vi "HW_Init.vi"(8 "error in":errorcluster, 9 "Traget FPS":i32=80, 10 "Close port? (T)":bool=TRUE, 11 "VISA resource name":refnum<visa-resource-name>="ASRL3::INSTR") -> (0 "error out":errorcluster, 1 "Sensors response":string="A1454", 2 "Instrument OK?":bool=TRUE, 3 "VISA resource name out":refnum<visa-resource-name>="ASRL3::INSTR", 4 "Sync mode status":string, 5 "Sensor board size":string, 6 "FPS status":i32=80, 7 "Version information":string)   [LabVIEW 2016]
uses:
  <vilib>/Utility/error.llb/DialogType.ctl
  <vilib>/Instr/_visa.llb/VISA Set IO Buffer Mask.ctl
  <vilib>/Instr/_visa.llb/VISA Flush IO Buffer Mask.ctl
  <vilib>/Instr/_visa.llb/VISA Configure Serial Port (Instr).vi
panel:
  out "Poll Sync mode status":u32
  out "Poll Port data status":u32
  out "Port data status":i32=1
  out "Latest Poll results (before implemented adjustments)":string="P\r\nI am alive!\r\nA1454 OK!\r\nBinary mode ON\r\nCoordinate mode ON\r\nMatrix mode OFF\r\nFPS target=80\r\nExternal USART status: 0\r\nLed status: 1\r\nPort data status: 1\r\nIOS: 1 = 0, 2 = 0 3 = 0, 4 = 0\r\nOK\r\n"
  out "Poll Binary":u32
  out "Poll Matrix":u32
  out "Poll Coord":u32
  out "Poll FPS":u32
  out "Matrix mode status":string="OFF"
  out "Coordinate mode status":string="ON"
  out "Binary mode status":string="ON"
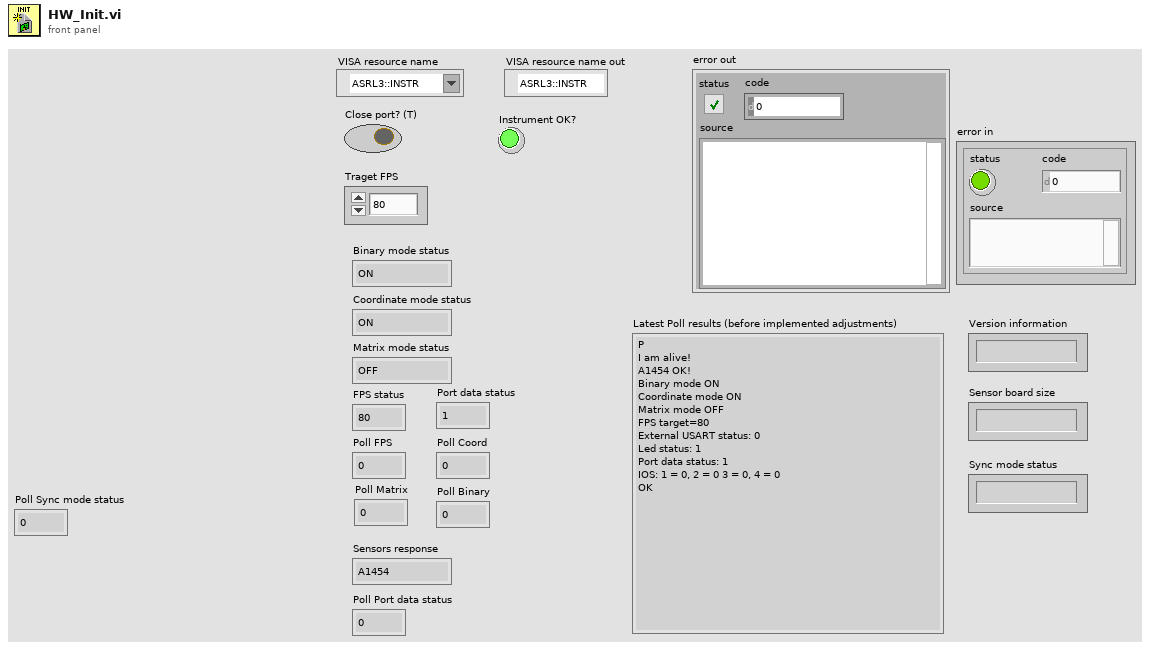
[diagram p1: front panel]
types:
  T1 = typedef "DialogType.ctl" = u16
  T2 = typedef "VISA Set IO Buffer Mask.ctl" = u16
  T3 = typedef "VISA Flush IO Buffer Mask.ctl" = u16
  T4 = cluster{"Matrix mode status":string, "Coordinate mode status":string, "Binary mode status":string, "Sensors response":string, "FPS status":i32, "Port data status":i32}
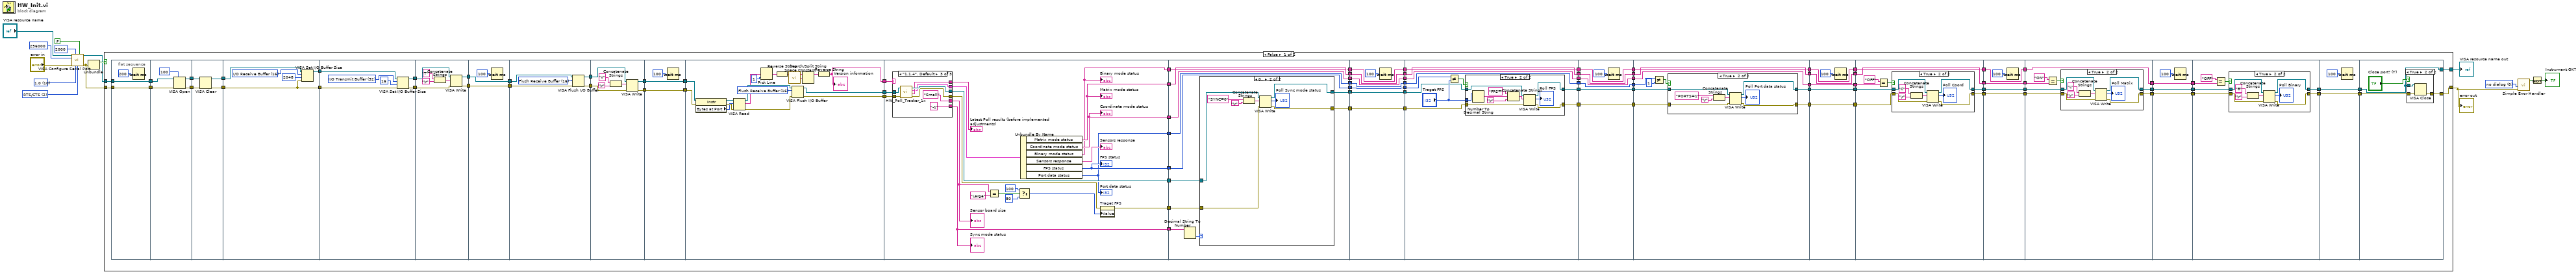
[diagram p0: block diagram]
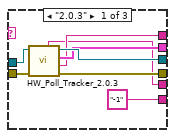
[diagram p2: hidden frame]
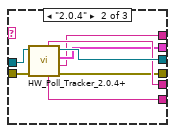
[diagram p3: hidden frame]
diagram:
  w1 = u16 10 items=["1.0"=10, "1.5"=15, "2.0"=20] ("stop bits (10: 1 bit)")
  w3 = T1 0 items=["no dialog", "OK message", "continue or stop message", "OK message + warnings", "continue/stop + warnings"] ("type of dialog (OK msg:1)")
  w9 = u16 2 items=["None", "XON/XOFF", "RTS/CTS", "XON/XOFF & RTS/CTS", "DTR/DSR", "XON/XOFF & DTR/DSR"] ("flow control (0:none)")
  n1 = call-poly "VISA Configure Serial Port"("VISA resource name"="VISA resource name", "timeout (10sec)"=u32 2000, "Enable Termination\nChar (T)"=FALSE ("Enable Termination\nChar (T)"), "baud rate (9600)"=u32 256000, "error in (no error)"="error in", "stop bits (10: 1 bit)"=w1, "flow control (0:none)"=w9) -> ("VISA resource name out"=w7:refnum<visa-resource-name>, "error out"=w11:errorcluster)  [unwired: 7 in]
  n2 = Unbundle(w11) -> ("status"=w10:bool)  [unwired: 2 out]
  n3 = case shown="False" w10 {
    tunnel: w7 -> [w73 w374]
    tunnel: w11 -> [w72 w375]
    tunnel: [w54 w375] -> w6
    tunnel: [w53 w374] -> w8
    frame False {
      n4 = flat-sequence {
        tunnel: [w106] -> w104
        tunnel: [w105] -> w103
        tunnel: w73 -> [w106]
        tunnel: w72 -> [w105]
        tunnel: w104 -> [w110]
        tunnel: [w109] -> w101
        tunnel: w103 -> [w112]
        tunnel: [w111] -> w102
        tunnel: w102 -> [w115]
        tunnel: w101 -> [w116]
        tunnel: [w114] -> w100
        tunnel: [w113] -> w99
        tunnel: [w117] -> w97
        tunnel: [w121] -> w98
        tunnel: w100 -> [w117]
        tunnel: w99 -> [w119]
        tunnel: w98 -> [w125]
        tunnel: [w124] -> w46
        tunnel: w97 -> [w123]
        tunnel: [w122] -> w45
        tunnel: w46 -> [w131]
        tunnel: [w129] -> w42
        tunnel: w45 -> [w130]
        tunnel: [w128] -> w40
        tunnel: w42 -> [w137]
        tunnel: [w137] -> w41
        tunnel: w40 -> [w136]
        tunnel: [w136] -> w39
        tunnel: w41 -> [w140]
        tunnel: [w139] -> w44
        tunnel: w39 -> [w142]
        tunnel: [w141] -> w43
        tunnel: w44 -> [w145]
        tunnel: w43 -> [w146]
        tunnel: [w144] -> w52
        tunnel: [w143] -> w51
        tunnel: w52 -> [w152]
        tunnel: [w152] -> w50
        tunnel: w51 -> [w151]
        tunnel: [w151] -> w48
        tunnel: w50 -> [w165]
        tunnel: [w163] -> w49
        tunnel: w48 -> [w166]
        tunnel: [w161] -> w47
        tunnel: [w153] -> w38
        tunnel: [w177] -> w29
        tunnel: [w190] -> w30
        tunnel: w49 -> [w188]
        tunnel: [w181] -> w27
        tunnel: [w184] -> w25
        tunnel: [w185] -> w23
        tunnel: [w183] -> w21
        tunnel: [w180] -> w19
        tunnel: w47 -> [w187]
        tunnel: w38 -> [w179]
        tunnel: [w170] -> w16
        tunnel: w30 -> [w220]
        tunnel: w29 -> [w218]
        tunnel: [w217] -> w28
        tunnel: w27 -> [w225]
        tunnel: [w225] -> w26
        tunnel: w25 -> [w224]
        tunnel: [w224] -> w24
        tunnel: w23 -> [w223]
        tunnel: [w223] -> w22
        tunnel: w21 -> [w222]
        tunnel: [w222] -> w20
        tunnel: w19 -> [w221]
        tunnel: [w221] -> w18
        tunnel: [w219] -> w17
        tunnel: w16 -> [w216]
        tunnel: [w243] -> w37
        tunnel: w28 -> [w242]
        tunnel: [w242] -> w36
        tunnel: w26 -> [w241]
        tunnel: [w241] -> w35
        tunnel: w24 -> [w240]
        tunnel: [w240] -> w34
        tunnel: w22 -> [w239]
        tunnel: [w239] -> w33
        tunnel: w20 -> [w238]
        tunnel: [w238] -> w32
        tunnel: w18 -> [w237]
        tunnel: [w237] -> w31
        tunnel: w17 -> [w243]
        tunnel: w37 -> [w252]
        tunnel: [w249] -> w96
        tunnel: w36 -> [w251]
        tunnel: [w250] -> w95
        tunnel: w35 -> [w253]
        tunnel: [w248] -> w94
        tunnel: w34 -> [w248]
        tunnel: [w247] -> w93
        tunnel: w33 -> [w247]
        tunnel: [w246] -> w92
        tunnel: w32 -> [w246]
        tunnel: w31 -> [w245]
        tunnel: [w245] -> w55
        tunnel: w96 -> [w273]
        tunnel: [w273] -> w71
        tunnel: w95 -> [w272]
        tunnel: [w272] -> w70
        tunnel: [w270] -> w69
        tunnel: w94 -> [w270]
        tunnel: [w269] -> w68
        tunnel: w93 -> [w269]
        tunnel: [w268] -> w67
        tunnel: w92 -> [w268]
        tunnel: [w267] -> w56
        tunnel: w55 -> [w267]
        tunnel: w71 -> [w278]
        tunnel: [w277] -> w66
        tunnel: w70 -> [w280]
        tunnel: [w279] -> w64
        tunnel: w69 -> [w283]
        tunnel: [w283] -> w62
        tunnel: w68 -> [w282]
        tunnel: [w282] -> w60
        tunnel: w67 -> [w281]
        tunnel: [w281] -> w58
        tunnel: w56 -> [w275]
        tunnel: w66 -> [w299]
        tunnel: [w299] -> w65
        tunnel: w64 -> [w298]
        tunnel: [w298] -> w63
        tunnel: w62 -> [w297]
        tunnel: [w297] -> w61
        tunnel: w60 -> [w296]
        tunnel: [w296] -> w59
        tunnel: w58 -> [w295]
        tunnel: [w295] -> w57
        tunnel: w65 -> [w307]
        tunnel: [w305] -> w91
        tunnel: w63 -> [w306]
        tunnel: [w302] -> w90
        tunnel: w61 -> [w304]
        tunnel: w59 -> [w301]
        tunnel: [w301] -> w89
        tunnel: w57 -> [w300]
        tunnel: [w300] -> w88
        tunnel: w91 -> [w323]
        tunnel: [w323] -> w87
        tunnel: w90 -> [w322]
        tunnel: [w322] -> w86
        tunnel: [w320] -> w85
        tunnel: w89 -> [w320]
        tunnel: [w319] -> w84
        tunnel: w88 -> [w319]
        tunnel: w87 -> [w329]
        tunnel: [w327] -> w83
        tunnel: w86 -> [w328]
        tunnel: [w326] -> w82
        tunnel: w85 -> [w325]
        tunnel: w84 -> [w324]
        tunnel: [w324] -> w81
        tunnel: w83 -> [w345]
        tunnel: [w345] -> w80
        tunnel: w82 -> [w344]
        tunnel: [w344] -> w79
        tunnel: [w342] -> w78
        tunnel: w81 -> [w342]
        tunnel: w80 -> [w350]
        tunnel: [w348] -> w77
        tunnel: w79 -> [w349]
        tunnel: [w347] -> w76
        tunnel: w78 -> [w346]
        tunnel: w77 -> [w365]
        tunnel: [w365] -> w75
        tunnel: [w364] -> w74
        tunnel: w76 -> [w364]
        tunnel: w75 -> [w366]
        tunnel: w74 -> [w369]
        tunnel: [w367] -> w54
        tunnel: [w366] -> w53
        frame #0 {
          n5 = Wait (ms)(milliseconds to wait=u32 200) -> ()  [unwired: 1 out]
        }
        frame #1 {
          n6 = VISA Open(timeout (0)=u32 100 ("VISA Open timeout (0)"), error in (no error)=w112, VISA resource name=w110) -> (VISA resource name=w109:refnum<visa-resource-name>, error out=w111:errorcluster)  [unwired: 2 in]
        }
        frame #2 {
          n7 = VISA Clear(VISA resource name=w116, error in (no error)=w115) -> (VISA resource name out=w113:refnum<visa-resource-name>, error out=w114:errorcluster)
        }
        frame #3 {
          w118 = T2 16 items=["I/O Receive Buffer"=16, "I/O Transmit Buffer"=32, "I/O Receive and Transmit Buffer"=48] ("Mask")
          n8 = VISA Set I/O Buffer Size(VISA resource name=w119, mask (16)=w118, size (4096)=u32 2048, error in (no error)=w117) -> (VISA resource name out=w121:refnum<visa-resource-name>)  [unwired: 1 out]
        }
        frame #4 {
          w126 = T2 32 items=["I/O Receive Buffer"=16, "I/O Transmit Buffer"=32, "I/O Receive and Transmit Buffer"=48] ("Mask")
          n9 = VISA Set I/O Buffer Size(VISA resource name=w125, mask (16)=w126, size (4096)=u32 16, error in (no error)=w123) -> (VISA resource name out=w124:refnum<visa-resource-name>, error out=w122:errorcluster)
        }
        frame #5 {
          n10 = Concatenate Strings("T" ("write buffer"), "\r") -> (w132:string)
          n11 = VISA Write(VISA resource name=w131, write buffer=w132, error in (no error)=w130) -> (VISA resource name out=w129:refnum<visa-resource-name>, error out=w128:errorcluster)  [unwired: 1 out]
        }
        frame #6 {
          n12 = Wait (ms)(milliseconds to wait=u32 100) -> ()  [unwired: 1 out]
        }
        frame #7 {
          w138 = T3 16 items=["Flush Receive Buffer"=16, "Write Transmit Buffer to Device"=32, "Flush Receive Buffer (No I/O)"=64, "Flush Transmit Buffer"=128] ("Mask")
          n13 = VISA Flush I/O Buffer(VISA resource name=w140, mask (16)=w138, error in (no error)=w142) -> (VISA resource name out=w139:refnum<visa-resource-name>, error out=w141:errorcluster)
        }
        frame #8 {
          n14 = Concatenate Strings("V" ("write buffer"), "\r") -> (w147:string)
          n15 = VISA Write(VISA resource name=w145, write buffer=w147, error in (no error)=w146) -> (VISA resource name out=w143:refnum<visa-resource-name>, error out=w144:errorcluster)  [unwired: 1 out]
        }
        frame #9 {
          n16 = Wait (ms)(milliseconds to wait=u32 100) -> ()  [unwired: 1 out]
        }
        frame #10 {
          w160 = T3 16 items=["Flush Receive Buffer"=16, "Write Transmit Buffer to Device"=32, "Flush Receive Buffer (No I/O)"=64, "Flush Transmit Buffer"=128] ("Mask")
          n17 = property class="Instr"(reference=w166, error in=w165) -> (reference out=w169:refnum<visa-resource-name>, error out=w168:errorcluster, "Bytes at Port"=w167:u32)
          n18 = VISA Read(VISA resource name=w169, byte count=w167, error in (no error)=w168) -> (VISA resource name out=w162:refnum<visa-resource-name>, read buffer=w159:string, error out=w164:errorcluster)  [unwired: 1 out]
          n19 = Pick Line(multi-line string=w159, line index=1) -> (output string=w157:string)  [unwired: 1 in]
          n20 = Reverse String(1:w157) -> (0:w156:string)
          n21 = call <vilib>:"Space Constant.vi"() -> ("String"=w155:string)
          n22 = VISA Flush I/O Buffer(VISA resource name=w162, mask (16)=w160, error in (no error)=w164) -> (VISA resource name out=w161:refnum<visa-resource-name>, error out=w163:errorcluster)
          n23 = Search/Split String(string=w156, search string/char (-)=w155) -> (substring before match=w154:string)  [unwired: 1 in, 2 out]
          n24 = Reverse String(1:w154) -> (0:w153:string)
          "Version information" <- w153
        }
        frame #11 {
          n25 = case shown="\"1.1.4\", Default" w179 {
            tunnel: [w195 w204 w214] -> w190
            tunnel: [w193 w201 w213] -> w189
            tunnel: w188 -> [w198 w205 w212]
            tunnel: w187 -> [w196 w206 w211]
            tunnel: [w197 w200 w210] -> w178
            tunnel: [w194 w202 w209] -> w186
            tunnel: [w192 w203 "Small"] -> w176
            tunnel: ["-1" ("Sync mode status") w199 "-1" ("Sync mode status")] -> w170
            frame "2.0.3" {
              n26 = call "HW_Poll_Tracker_2.0.3.vi"("error in"=w198, "VISA resource name in"=w196) -> ("error out"=w197:errorcluster, "Read buffer"=w193:string, "Parameters output"=w194:T4, "VISA resource name out"=w195:refnum<visa-resource-name>, "Sensor board size"=w192:string)  [unwired: 5 in]
            }
            frame "2.0.4" {
              n27 = call "HW_Poll_Tracker_2.0.4+.vi"("error in"=w205, "VISA resource name in"=w206) -> ("error out"=w200:errorcluster, "Read buffer"=w201:string, "Parameters output"=w202:T4, "VISA resource name out"=w204:refnum<visa-resource-name>, "Sync mode status"=w199:string, "Sensor board size"=w203:string)  [unwired: 4 in]
            }
            frame "1.1.4", Default {
              n28 = call "HW_Poll_Tracker_1x.vi"("error in"=w212, "VISA resource name in"=w211) -> ("error out"=w210:errorcluster, "Read buffer"=w213:string, "Parameters output"=w209:T4, "VISA resource name out"=w214:refnum<visa-resource-name>)  [unwired: 6 in]
            }
          }
          "Latest Poll results (before implemented adjustments)" <- w189
          "Sensor board size" <- w176
          "Sync mode status" <- w170
          n29 = Equal?(x=w176, y="Large") -> (x = y?=w174:bool)
          n30 = Select(t=100, s=w174, f=80) -> (s? t:f=w171:i32)
          n31 = Unbundle By Name(w186) -> ("Matrix mode status"=w185:string, "Coordinate mode status"=w184:string, "Binary mode status"=w183:string, "Sensors response"=→"Sensors response":string, "FPS status"=w181:i32, "Port data status"=w180:i32)
          "Binary mode status" <- w183
          "Coordinate mode status" <- w184
          "Matrix mode status" <- w185
          "FPS status" <- w181
          "Port data status" <- w180
          n32 = property on="Traget FPS" class="DigNum (strict)"(error in=w178, "Value"=w171) -> (error out=w177:errorcluster)  [unwired: 1 in, 1 out]
        }
        frame #12 {
          n33 = Decimal String To Number(string=w216) -> (number=w215:i32)  [unwired: 2 in, 1 out]
          n34 = case shown="0.." w215 {
            tunnel: w220 -> [w227 w233]
            tunnel: w218 -> [w226 w232]
            tunnel: [w226 w231] -> w217
            tunnel: [w227 w230] -> w219
            frame -1, Default {
            }
            frame 0.. {
              n35 = Concatenate Strings("SYNC=0" ("write buffer"), "\r") -> (w235:string)
              n36 = VISA Write(VISA resource name=w233, write buffer=w235, error in (no error)=w232) -> (VISA resource name out=w230:refnum<visa-resource-name>, return count=→"Poll Sync mode status":u32, error out=w231:errorcluster)
            }
          }
        }
        frame #13 {
          n37 = Wait (ms)(milliseconds to wait=u32 100) -> ()  [unwired: 1 out]
        }
        frame #14 {
          n38 = Not Equal?(x=w253, y="Traget FPS") -> (x != y?=w254:bool)
          n39 = case shown="True" w254 {
            tunnel: w252 -> [w256 w263]
            tunnel: w251 -> [w255 w262]
            tunnel: [w255 w261] -> w250
            tunnel: [w256 w260] -> w249
            tunnel: "Traget FPS" -> [_ w258]
            frame False {
            }
            frame True {
              n40 = Number To Decimal String(number=w258) -> (decimal integer string=w257:string)  [unwired: 1 in]
              n41 = Concatenate Strings("FPS=" ("write buffer"), w257, "\r") -> (w265:string)
              n42 = VISA Write(VISA resource name=w263, write buffer=w265, error in (no error)=w262) -> (VISA resource name out=w260:refnum<visa-resource-name>, return count=→"Poll FPS":u32, error out=w261:errorcluster)
            }
          }
        }
        frame #15 {
          n43 = Wait (ms)(milliseconds to wait=u32 100) -> ()  [unwired: 1 out]
        }
        frame #16 {
          n44 = Not Equal?(x=w275, y=1) -> (x != y?=w274:bool)
          n45 = case shown="True" w274 {
            tunnel: w280 -> [w284 w289]
            tunnel: [w284 w288] -> w279
            tunnel: w278 -> [w285 w287]
            tunnel: [w285 w286] -> w277
            frame False {
            }
            frame True {
              n46 = Concatenate Strings("PORTS=1" ("write buffer"), "\r") -> (w291:string)
              n47 = VISA Write(VISA resource name=w287, write buffer=w291, error in (no error)=w289) -> (VISA resource name out=w286:refnum<visa-resource-name>, return count=→"Poll Port data status":u32, error out=w288:errorcluster)
            }
          }
        }
        frame #17 {
          n48 = Wait (ms)(milliseconds to wait=u32 100) -> ()  [unwired: 1 out]
        }
        frame #18 {
          n49 = Equal?(x="OFF", y=w304) -> (x = y?=w308:bool)
          n50 = case shown="True" w308 {
            tunnel: w307 -> [w310 w314]
            tunnel: w306 -> [w309 w313]
            tunnel: [w310 w312] -> w305
            tunnel: [w309 w311] -> w302
            frame False {
            }
            frame True {
              n51 = Concatenate Strings("C" ("write buffer"), "\r") -> (w316:string)
              n52 = VISA Write(VISA resource name=w314, write buffer=w316, error in (no error)=w313) -> (VISA resource name out=w312:refnum<visa-resource-name>, return count=→"Poll Coord":u32, error out=w311:errorcluster)
            }
          }
        }
        frame #19 {
          n53 = Wait (ms)(milliseconds to wait=u32 100) -> ()  [unwired: 1 out]
        }
        frame #20 {
          n54 = Equal?(x="ON", y=w325) -> (x = y?=w331:bool)
          n55 = case shown="True" w331 {
            tunnel: w329 -> [w333 w337]
            tunnel: w328 -> [w332 w336]
            tunnel: [w333 w335] -> w327
            tunnel: [w332 w334] -> w326
            frame False {
            }
            frame True {
              n56 = Concatenate Strings("L" ("write buffer"), "\r") -> (w339:string)
              n57 = VISA Write(VISA resource name=w337, write buffer=w339, error in (no error)=w336) -> (VISA resource name out=w335:refnum<visa-resource-name>, return count=→"Poll Matrix":u32, error out=w334:errorcluster)
            }
          }
        }
        frame #21 {
          n58 = Wait (ms)(milliseconds to wait=u32 100) -> ()  [unwired: 1 out]
        }
        frame #22 {
          n59 = Equal?(x="OFF", y=w346) -> (x = y?=w352:bool)
          n60 = case shown="True" w352 {
            tunnel: w350 -> [w354 w358]
            tunnel: w349 -> [w353 w357]
            tunnel: [w354 w356] -> w348
            tunnel: [w353 w355] -> w347
            frame False {
            }
            frame True {
              n61 = Concatenate Strings("B" ("write buffer"), "\r") -> (w360:string)
              n62 = VISA Write(VISA resource name=w358, write buffer=w360, error in (no error)=w357) -> (VISA resource name out=w356:refnum<visa-resource-name>, return count=→"Poll Binary":u32, error out=w355:errorcluster)
            }
          }
        }
        frame #23 {
          n63 = Wait (ms)(milliseconds to wait=u32 100) -> ()  [unwired: 1 out]
        }
        frame #24 {
          n64 = case shown="True" "Close port? (T)" {
            tunnel: w369 -> [w370 w373]
            tunnel: [w370 w372] -> w367
            tunnel: w366 -> [_ w371]
            frame False {
            }
            frame True {
              n65 = VISA Close(VISA resource name=w371, error in (no error)=w373) -> (error out=w372:errorcluster)
            }
          }
        }
      }
    }
    frame True {
    }
  }
  "error out" <- w6
  "VISA resource name out" <- w8
  n66 = call <vilib>:"Simple Error Handler.vi"("type of dialog (OK msg:1)"=w3, "error in (no error)"=w6) -> ("error?"=w5:bool)  [unwired: 3 in, 4 out]
  n67 = Not(x=w5) -> (.not. x?=→"Instrument OK?":bool)
